vi "PCO_LoadPseudoLut.vi"(8 "error in (no error)":errorcluster {"code" format="%x"}, 9 "filename":string, 10 "format":i32, 11 "ph":u64) -> (0 "error out":errorcluster {"code" format="%x"}, 2 "ErrorMessage":i32 format="%x", 3 "ph out":u64)   [LabVIEW 2019, in "Convert.lvlib"]
doc: "int PCOCONVERT_API PCO_LoadPseudoLut(HANDLE ph, int format, char *filename);"
uses:
  Convert.lvlib
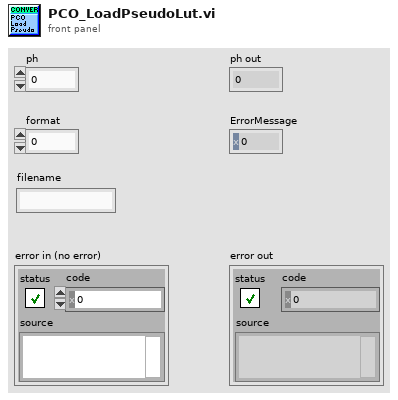
[diagram p1: front panel]
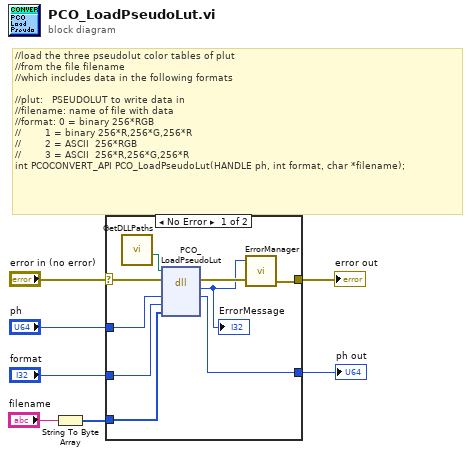
[diagram p0: block diagram]
diagram:
  # "//load the three pseudolut color tables of plut\n//from the file filename\n//which includes data in the following formats\n\n//plut:   PSEUDOLUT to write data in \n//filename: name of file with data\n//format: 0 = binary 256*RGB\n//        1 = binary 256*R,256*G,256*R\n//        2 = ASCII  256*RGB \n//        3 = ASCII  256*R,256*G,256*R\nint PCOCONVERT_API PCO_LoadPseudoLut(HANDLE ph, int format, char *filename);"
  n1 = String To Byte Array(string="filename") -> (unsigned byte array=w1:u8[])
  n2 = case shown="No Error" "error in (no error)" {
    selector: "error in (no error)" -> [w9 w18]
    tunnel: "ph" -> [w16 w17]
    tunnel: [w15 w17] -> w6
    tunnel: "format" -> [w14 _]
    tunnel: w1 -> [w13 _]
    tunnel: [w11 w18] -> w4
    frame No Error {
      n3 = call "GetDLLPaths.vi"() -> ("PCO_Conv_Path"=w8:path)  [unwired: 9 in, 2 out]
      n4 = dll-call lib="?" fn="PCO_LoadPseudoLut"(path in=w8, error in=w9, "ph"=w16, "format"=w14, "filename"=w13) -> (error out=w12:errorcluster, "return type"=w10:i32, "ph"=w15:u64)  [unwired: 3 in, 1 out]
      "ErrorMessage" <- w10
      n5 = call "ErrorManager.vi"("error in (no error)"=w12, "error code"=w10) -> ("error out"=w11:errorcluster)  [unwired: 3 in]
    }
    frame Error {
    }
  }
  "ph out" <- w6
  "error out" <- w4
